vi "UI Initialize.vi"(8 "error in (no error)":errorcluster, 11 "View in":refnum<class "MCListbox View.lvclass">) -> (0 "error out":errorcluster, 3 "View out":refnum<class "MCListbox View.lvclass">)   [LabVIEW 2013, in "SET Project Editor.lvlib" / "MCListbox View.lvclass"]
uses:
  MCListbox View.lvclass
  <vilib>/Utility/miscctls.llb/LVRowAndColumnTypeDef.ctl
  MCListbox View.lvclass/MCListbox View.ctl
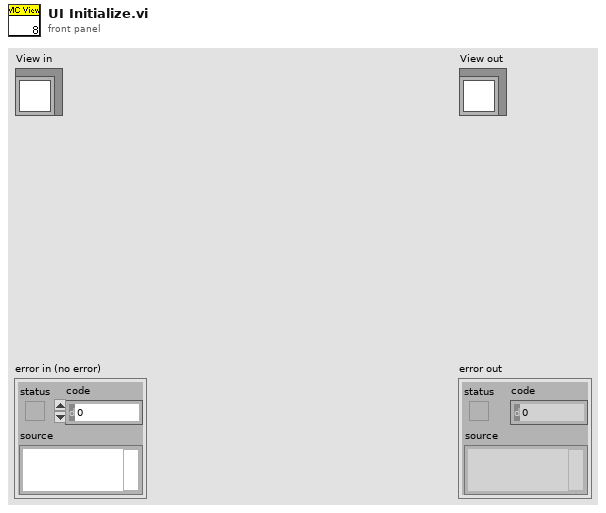
[diagram p1: front panel]
types:
  T1 = typedef "LVRowAndColumnTypeDef.ctl" = cluster{"Row":i32, "Column":i32}
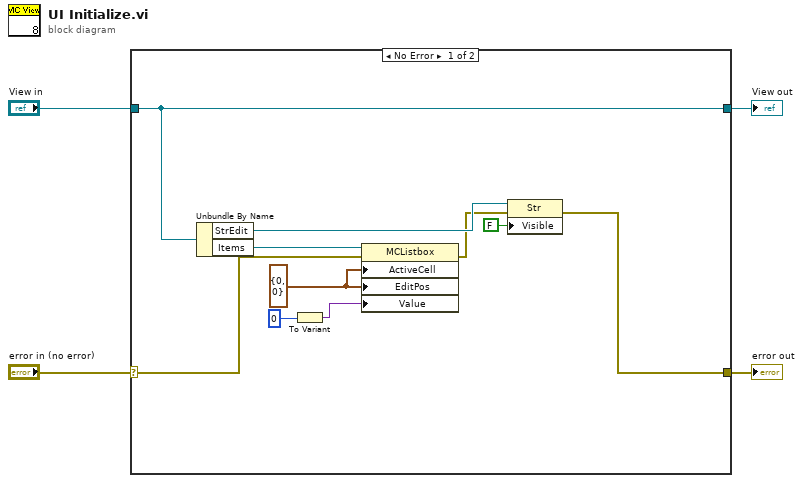
[diagram p0: block diagram]
diagram:
  n1 = case shown="No Error" "error in (no error)" {
    selector: "error in (no error)" -> [w6 w16]
    tunnel: [w5 w16] -> w3
    tunnel: [w14 w15] -> w1
    tunnel: "View in" -> [w14 w15]
    frame No Error {
      w10 = T1 {"Row"=0, "Column"=0} ("Active Cell:Active Cell")
      n2 = Unbundle By Name(w14) -> ("StrEdit"=w13:refnum<vi>, "Items"=w11:refnum<vi>)
      n3 = To Variant(anything=0) -> (Variant=w8:variant)
      n4 = property class="MCListbox"(reference=w11, error in=w6, "ActiveCell"=w10, "EditPos"=w10, "Value"=w8) -> (error out=w7:errorcluster)  [unwired: 1 out]
      n5 = property class="Str"(reference=w13, error in=w7, "Visible"=FALSE) -> (error out=w5:errorcluster)  [unwired: 1 out]
    }
    frame Error {
    }
  }
  "error out" <- w3
  "View out" <- w1
